vi "FindAddresses.vi"(0 "_Driver_interaction in":refnum<class "_Driver_interaction.lvclass">, 3 "error in (no error)":errorcluster) -> (7 "_Driver_interaction out":refnum<class "_Driver_interaction.lvclass">, 8 "Devices_Addressed":i32, 10 "error out":errorcluster)   [LabVIEW 2014, in "Driver_interaction.lvlib" / "_Driver_interaction.lvclass"]
uses:
  _Driver_interaction.lvclass
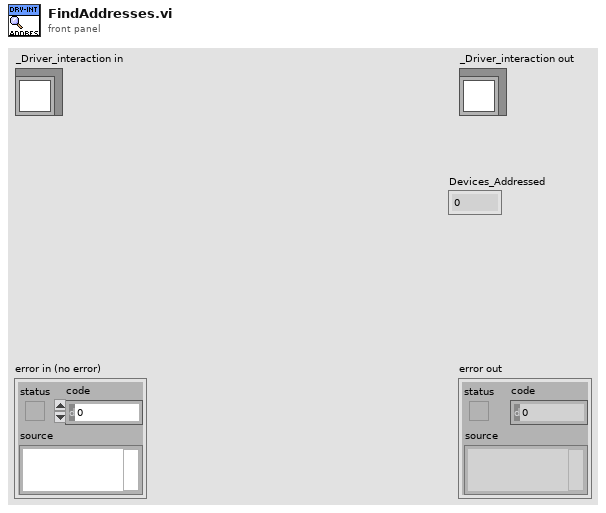
[diagram p1: front panel]
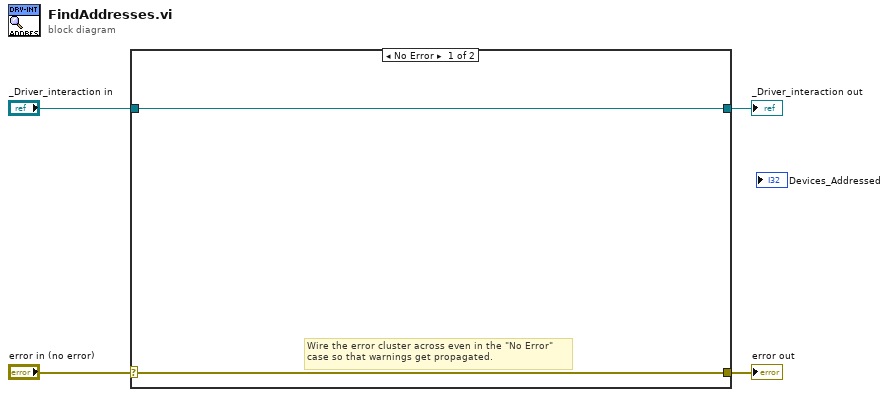
[diagram p0: block diagram]
diagram:
  n1 = case shown="No Error" "error in (no error)" {
    selector: "error in (no error)" -> [w5 w8]
    tunnel: [w5 w8] -> w3
    tunnel: [w6 w7] -> w1
    tunnel: "_Driver_interaction in" -> [w6 w7]
    frame No Error {
      # "Wire the error cluster across even in the \"No Error\"\ncase so that warnings get propagated."
    }
    frame Error {
    }
  }
  "error out" <- w3
  "_Driver_interaction out" <- w1
